vi "p2.vi"() -> ()   [LabVIEW 2023, in "d20.lvlib"]
uses:
  d20.lvlib
  Module Type.ctl
  AOC/AOC.lvlib
  d8/d8.lvlib
panel:
  in  "Example":string
  in  "Example":bool=TRUE
  out "Answer":u64
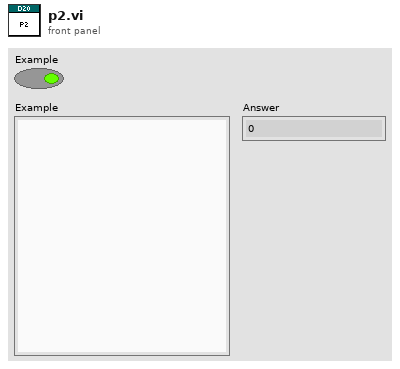
[diagram p1: front panel]
types:
  T1 = typedef "d20.lvlib/Module Type.ctl" = enum16{"broadcaster", "flip-flop", "conjunction", "output"}
  T2 = cluster{"Module Type":T1, "States":bool[], "Destinations":string[], "Sources":string[]}
  T3 = cluster{"Module Type":T1, "States":bool[], "string array":string[], "string array 2":string[]}
  T4 = map{string, cluster{"Module Type":T1, "States":bool[], "Destinations":string[], "Sources":string[]}}
  T5 = cluster{"Module Type":T1, "States":bool[], "string array":string[], "substring before match":string[]}
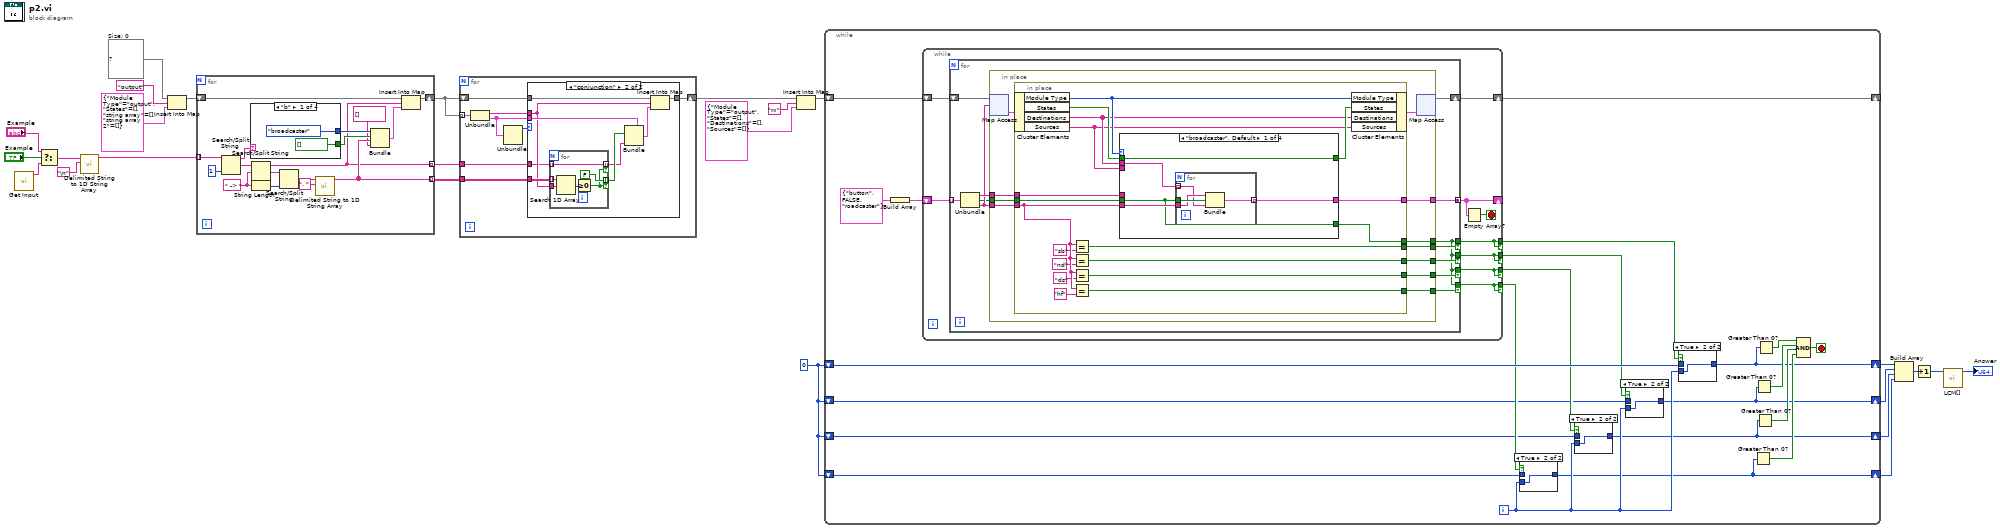
[diagram p0: block diagram]
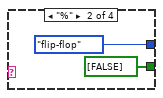
[diagram p3: hidden frame]
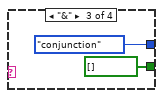
[diagram p4: hidden frame]
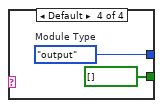
[diagram p5: hidden frame]
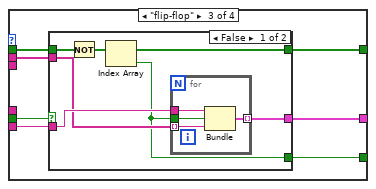
[diagram p11: hidden frame]
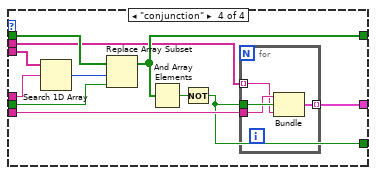
[diagram p13: hidden frame]
diagram:
  w8 = u64 0
  w19 = T4 {}  # Size: 0
  n1 = call "Get Input.vi"() -> ("Input"=w25:string)  [unwired: 11 in]
  n2 = Select(t="Example", s="Example", f=w25) -> (s? t:f=w22:string)
  n3 = call <vilib>:"Delimited String to 1D String Array.vi"("delimiter"="\n", "delimited string"=w22) -> ("string array"=w20:string[])  [unwired: 9 in]
  n4 = Insert Into Map(map in=w19, key="output", value=T3 {"Module Type"=enum."output", "States"=[], "string array"=[], "string array 2"=[]} ("output cluster")) -> (map out=w18:T4)  [unwired: 2 out]
  n5 = for {
    tunnel: w20 -> [w42] mode=indexing
    shift-right: [w39] -> w13
    shift-left: w18 -> [w38]
    tunnel: [w28] -> w15 mode=indexing
    tunnel: [w26] -> w14 mode=indexing
    w32 = " -> " ("search string/char (-)")
    n6 = Search/Split String(string=w42, offset (0)=1) -> (substring before match=w37:string, match + rest of string=w40:string)  [unwired: 1 in, 1 out]
    n7 = case shown="\"b\"" w37 {
      tunnel: [Module_Type."broadcaster" Module_Type."flip-flop" Module_Type."conjunction" w50] -> w36
      tunnel: [bool[] [] ("States") bool[] [FALSE] ("States") bool[] [] ("States") bool[] [] ("States")] -> w29
      frame "b" {
      }
      frame "%" {
      }
      frame "&" {
      }
      frame Default {
        w50 = Module_Type."output"  # Module Type
      }
    }
    n8 = Search/Split String(string=w40, search string/char (-)=w32) -> (substring before match=w26:string, match + rest of string=w34:string)  [unwired: 1 in, 1 out]
    n9 = String Length(string=w32) -> (length=w33:i32)
    n10 = Search/Split String(string=w34, offset (0)=w33) -> (match + rest of string=w31:string)  [unwired: 1 in, 2 out]
    n11 = call <vilib>:"Delimited String to 1D String Array.vi"("delimiter"=", ", "delimited string"=w31) -> ("string array"=w28:string[])  [unwired: 9 in]
    n12 = Bundle("Module Type"=w36, "States"=w29, "string array"=w28, "substring before match"=string[] []) -> (w35:T5)  [unwired: 1 in]
    n13 = Insert Into Map(map in=w38, key=w26, value=w35) -> (map out=w39:T4)  [unwired: 2 out]
  }
  n14 = for {
    shift-right: [w54] -> w10
    shift-left: w13 -> [w58]
    tunnel: w13 -> [w57] mode=indexing
    tunnel: w15 -> [w53]
    tunnel: w14 -> [w51]
    n15 = Unbundle(w57) -> (w56:string, "output cluster"=w52:T2)
    n16 = Unbundle(w52) -> ("Module Type"=w55:T1)  [unwired: 3 out]
    n17 = case shown="\"conjunction\"" w55 {
      tunnel: w58 -> [w59 w68]
      tunnel: w56 -> [_ w63]
      tunnel: [w59 w67] -> w54
      tunnel: w53 -> [_ w64]
      tunnel: w52 -> [_ w66]
      tunnel: w51 -> [_ w61]
      frame Default {
      }
      frame "conjunction" {
        n18 = for {
          tunnel: w64 -> [w72] mode=indexing
          tunnel: w63 -> [w71]
          tunnel: [FALSE] -> w62 mode=indexing if=w69
          tunnel: w61 -> [w70] mode=indexing
          tunnel: [w70] -> w60 mode=indexing if=w69
          n19 = Search 1D Array(1D array=w72, element=w71) -> (index of element=w73:i32)  [unwired: 1 in]
          n20 = Greater Or Equal To 0?(x=w73) -> (x >= 0?=w69:bool)
        }
        n21 = Bundle(cluster=w66, "States"=w62, "Sources"=w60) -> (w65:T2)  [unwired: 2 in]
        n22 = Insert Into Map(map in=w68, key=w63, value=w65) -> (map out=w67:T4)  [unwired: 2 out]
      }
    }
  }
  n23 = Insert Into Map(map in=w10, key="rx", value=T2 {"Module Type"=enum."output", "States"=[], "Destinations"=[], "Sources"=[]}) -> (map out=w9:T4)  [unwired: 2 out]
  n24 = while {
    shift-right: [w93] -> _
    shift-left: w9 -> [w94]
    shift-right: [w78] -> w7
    shift-left: w8 -> [w89]
    shift-right: [w77] -> w6
    shift-left: w8 -> [w83]
    shift-right: [w76] -> w5
    shift-left: w8 -> [w82]
    shift-right: [w75] -> w4
    shift-left: w8 -> [w81]
    i -> [w88]
    stop <- w80 stop-if-true
    n25 = Build Array(cluster{string, bool, string} {"button", FALSE, "roadcaster"}) -> (w95:cluster{string, bool, string}[])
    n26 = while {
      shift-right: [w112] -> w93
      shift-left: w94 -> [w113]
      shift-right: [w109] -> _
      shift-left: w95 -> [w110]
      tunnel: [w108] -> w87 if=w108
      tunnel: [w107] -> w86 if=w107
      tunnel: [w106] -> w85 if=w106
      tunnel: [w105] -> w84 if=w105
      stop <- w111 stop-if-true
      n27 = for {
        shift-right: [w122] -> w112
        shift-left: w113 -> [w125]
        tunnel: w110 -> [w124] mode=indexing
        tunnel: [w123] -> w109 mode=concatenating
        tunnel: [w115] -> w108 if=w118
        tunnel: [w115] -> w107 if=w117
        tunnel: [w115] -> w106 if=w116
        tunnel: [w115] -> w105 if=w114
        n28 = Unbundle(w124) -> (w121:string, w119:bool, w120:string)
        n29 = in-place {
          in-place-border: w119 -> [w136]
          in-place-border: [w135] -> w123
          in-place-border: w121 -> [w132]
          in-place-border: w120 -> [w131]
          in-place-border: [w130] -> w115
          in-place-border: [w129] -> w118
          in-place-border: [w128] -> w117
          in-place-border: [w127] -> w116
          in-place-border: [w126] -> w114
          n30 = in-place-map #1(w125, w120) -> (w134:T2)  [unwired: 1 in, 1 out]
          n31 = in-place {
            in-place-border: w136 -> [w146]
            in-place-border: [w154] -> w135
            in-place-border: w132 -> [w148]
            in-place-border: w131 -> [w147]
            in-place-border: [w145] -> w130
            in-place-border: [w137] -> w129
            in-place-border: [w138] -> w128
            in-place-border: [w139] -> w127
            in-place-border: [w140] -> w126
            n32 = in-place-cluster #2(w134) -> ("Module Type"=w152:T1, "States"=w153:bool[], "Destinations"=w150:string[], "Sources"=w149:string[])
            n33 = Equal?(x=w147, y="sb") -> (x = y?=w137:bool)
            n34 = Equal?(x=w147, y="nd") -> (x = y?=w138:bool)
            n35 = Equal?(x=w147, y="ds") -> (x = y?=w139:bool)
            n36 = Equal?(x=w147, y="hf") -> (x = y?=w140:bool)
            n37 = case shown="\"broadcaster\", Default" w152 {
              tunnel: w146 -> [w155 _ w166 w186]
              tunnel: [w159 _ w168 w192] -> w154
              tunnel: w150 -> [w156 _ w170 w185]
              tunnel: w153 -> [w158 w164 w171 w189]
              tunnel: [w158 w164 w169 w188] -> w151
              tunnel: w149 -> [_ _ _ w191]
              tunnel: w148 -> [_ _ _ w190]
              tunnel: w147 -> [w157 _ w167 w184]
              tunnel: [w155 _ w165 w183] -> w145
              frame "broadcaster", Default {
                n38 = for {
                  tunnel: w156 -> [w160] mode=indexing
                  tunnel: w155 -> [w163]
                  tunnel: [w162] -> w159 mode=indexing
                  tunnel: w157 -> [w161]
                  n39 = Bundle(w161, w163, "String"=w160) -> (w162:cluster{string, bool, "String":string})  [unwired: 1 in]
                }
              }
              frame "output" {
              }
              frame "flip-flop" {
                n40 = case shown="False" w166 {
                  tunnel: w171 -> [w177 w182]
                  tunnel: w170 -> [w173 _]
                  tunnel: [w176 w182] -> w169
                  tunnel: [w175 _] -> w168
                  tunnel: w167 -> [w174 _]
                  tunnel: [w172 _] -> w165
                  frame False {
                    n41 = Not(x=w177) -> (.not. x?=w176:bool[])
                    n42 = Index Array(array=w176) -> (element=w172:bool)  [unwired: 1 in]
                    n43 = for {
                      tunnel: w173 -> [w178] mode=indexing
                      tunnel: w172 -> [w181]
                      tunnel: [w180] -> w175 mode=indexing
                      tunnel: w174 -> [w179]
                      n44 = Bundle(w179, "Boolean"=w181, "String"=w178) -> (w180:cluster{string, "Boolean":bool, "String":string})  [unwired: 1 in]
                    }
                  }
                  frame True {
                  }
                }
              }
              frame "conjunction" {
                n45 = Search 1D Array(1D array=w191, element=w190) -> (index of element=w187:i32)  [unwired: 1 in]
                n46 = Replace Array Subset(array=w189, new element=w186, index=w187) -> (w188:bool[])
                n47 = And Array Elements(Boolean array=w188) -> (logical AND=w193:bool)
                n48 = Not(x=w193) -> (.not. x?=w183:bool)
                n49 = for {
                  tunnel: w185 -> [w194] mode=indexing
                  tunnel: w183 -> [w197]
                  tunnel: [w196] -> w192 mode=indexing
                  tunnel: w184 -> [w195]
                  n50 = Bundle(w195, w197, "String"=w194) -> (w196:cluster{string, bool, "String":string})  [unwired: 1 in]
                }
              }
            }
            n51 = in-place-cluster #2("Module Type"=w152, "States"=w151, "Destinations"=w150, "Sources"=w149) -> (w133:T2)
          }
          n52 = in-place-map #1(w133) -> (w122:T4)  [unwired: 1 in, 2 out]
        }
      }
      n53 = Empty Array?(array=w109) -> (empty?=w111:bool)
    }
    n54 = case shown="True" w84 {
      tunnel: w88 -> [_ w98]
      tunnel: w81 -> [w97 _]
      tunnel: [w97 w98] -> w75
      frame False {
      }
      frame True {
      }
    }
    n55 = case shown="True" w85 {
      tunnel: w88 -> [_ w100]
      tunnel: w82 -> [w99 _]
      tunnel: [w99 w100] -> w76
      frame False {
      }
      frame True {
      }
    }
    n56 = case shown="True" w86 {
      tunnel: w88 -> [_ w102]
      tunnel: w83 -> [w101 _]
      tunnel: [w101 w102] -> w77
      frame False {
      }
      frame True {
      }
    }
    n57 = case shown="True" w87 {
      tunnel: w88 -> [_ w104]
      tunnel: w89 -> [w103 _]
      tunnel: [w103 w104] -> w78
      frame False {
      }
      frame True {
      }
    }
    n58 = Greater Than 0?(x=w75) -> (x > 0?=w90:bool)
    n59 = Greater Than 0?(x=w77) -> (x > 0?=w92:bool)
    n60 = Greater Than 0?(x=w76) -> (x > 0?=w91:bool)
    n61 = Greater Than 0?(x=w78) -> (x > 0?=w79:bool)
    n62 = Compound Arithmetic op=AND(w79, w92, w91, w90) -> (w80:bool)
  }
  n63 = Build Array(w7, w6, w5, w4) -> (w3:u64[])
  n64 = Increment(x=w3) -> (x+1=w1:u64[])
  n65 = call "LCM[].vi"("Array"=w1) -> ("LCM"=→"Answer":u64)  [unwired: 10 in]
